vi "GUI Open Login.vi"(8 "error in (no error)":errorcluster, 11 "FOFB-Controller IP Address in":string) -> (0 "error out":errorcluster, 1 "Cancelled?":bool, 2 "Password":string, 3 "FOFB-Controller IP Address out":string)   [LabVIEW 2011, in "User Interface VIs.lvlib"]
uses:
  User Interface VIs.lvlib
  User Interface Window VIs.lvlib
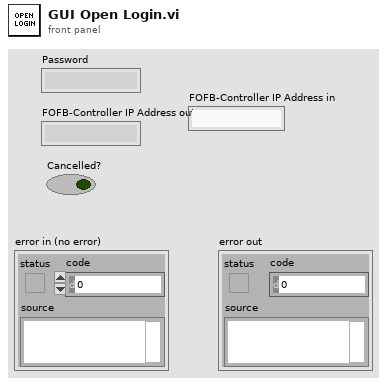
[diagram p1: front panel]
types:
  T1 = enum32{"Invalid", "Standard", "Closed", "Hidden", "Minimized", "Maximized"}
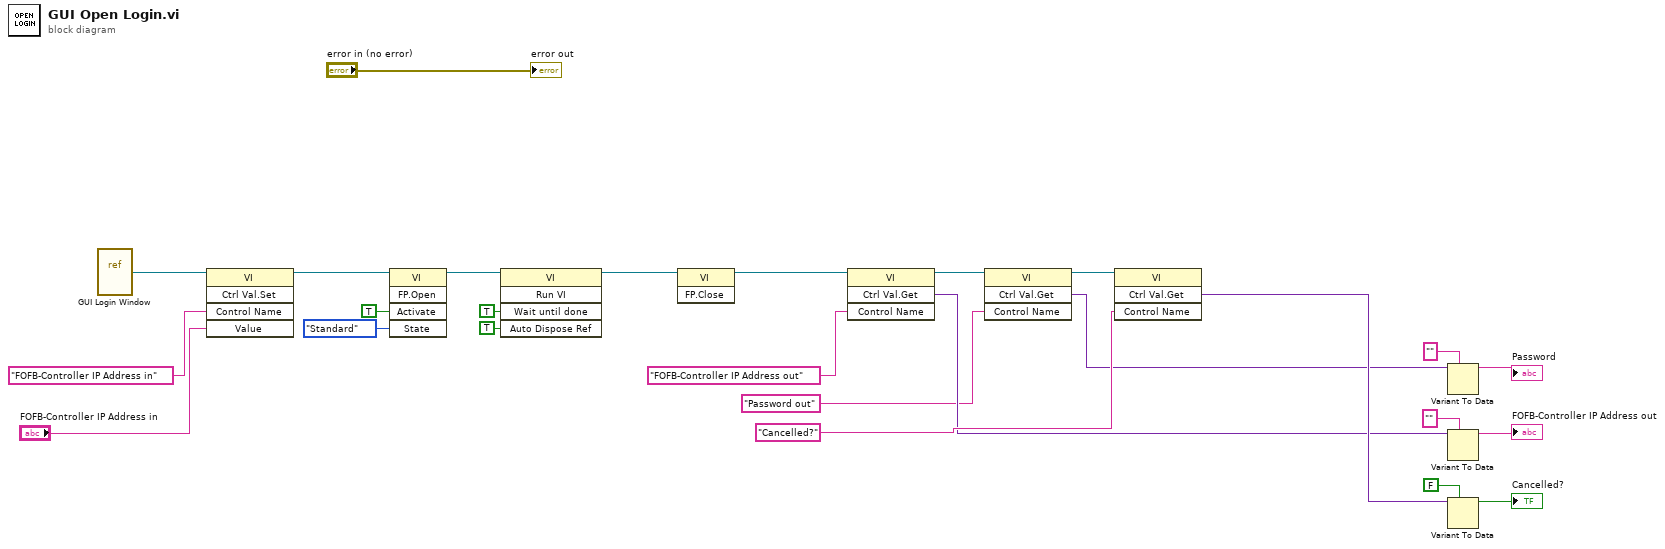
[diagram p0: block diagram]
diagram:
  n1 = vi-ref "GUI Login Window.vi"() -> (w26:refnum<vi>)
  n2 = invoke class="VI" method="Ctrl Val.Set"(reference=w26, "Control Name"="FOFB-Controller IP Address in", "Value"="FOFB-Controller IP Address in") -> (reference out=w11:refnum<vi>)  [unwired: 2 in, 4 out]
  n3 = invoke class="VI" method="FP.Open"(reference=w11, "Activate"=TRUE ("Activate?"), "State"=T1."Standard") -> (reference out=w4:refnum<vi>)  [unwired: 2 in, 4 out]
  n4 = invoke class="VI" method="Run VI"(reference=w4, "Wait until done"=TRUE ("Wait Until Done"), "Auto Dispose Ref"=TRUE ("Auto Dispose Reference")) -> (reference out=w3:refnum<vi>)  [unwired: 2 in, 4 out]
  n5 = invoke class="VI" method="FP.Close"(reference=w3) -> (reference out=w2:refnum<vi>)  [unwired: 2 in, 2 out]
  n6 = invoke class="VI" method="Ctrl Val.Get"(reference=w2, "Control Name"="FOFB-Controller IP Address out") -> (reference out=w12:refnum<vi>, "Get Control Value Variant"=w15:variant)  [unwired: 2 in, 2 out]
  n7 = invoke class="VI" method="Ctrl Val.Get"(reference=w12, "Control Name"="Password out") -> (reference out=w20:refnum<vi>, "Get Control Value Variant"=w16:variant)  [unwired: 2 in, 2 out]
  n8 = invoke class="VI" method="Ctrl Val.Get"(reference=w20, "Control Name"="Cancelled?") -> ("Get Control Value Variant"=w24:variant)  [unwired: 2 in, 3 out]
  n9 = Variant To Data(type="" ("Control Name"), Variant=w16) -> (data=→"Password":string)  [unwired: 1 in, 1 out]
  n10 = Variant To Data(type="" ("Control Name"), Variant=w15) -> (data=→"FOFB-Controller IP Address out":string)  [unwired: 1 in, 1 out]
  n11 = Variant To Data(type=FALSE ("Stop?"), Variant=w24) -> (data=→"Cancelled?":bool)  [unwired: 1 in, 1 out]
  "error out" <- "error in (no error)"
